vi "wrap.PullString.vi"(0 "class.GLue in":refnum<class "class.GLue.lvclass">, 11 "error in (no error)":errorcluster, 13 "Index":i32=-1) -> (4 "class.GLue out":refnum<class "class.GLue.lvclass">, 8 "String":string, 15 "error out":errorcluster)   [LabVIEW 2014, in "GLue.lvlib" / "class.GLue.lvclass"]
uses:
  class.GLue.lvclass
  class.GLue.lvclass/class.GLue.ctl
  Resources/GLue.dll
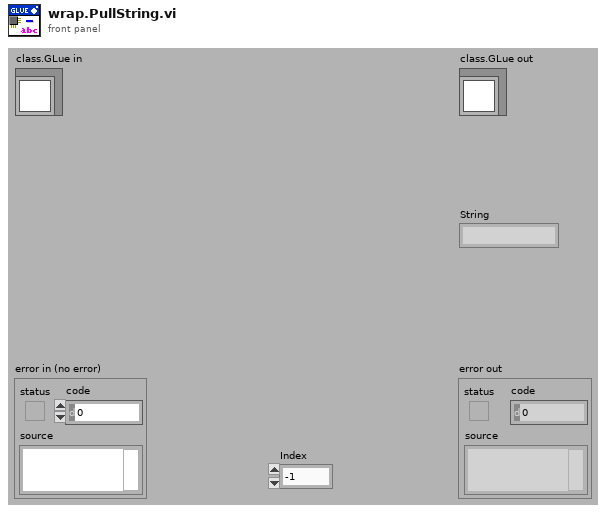
[diagram p1: front panel]
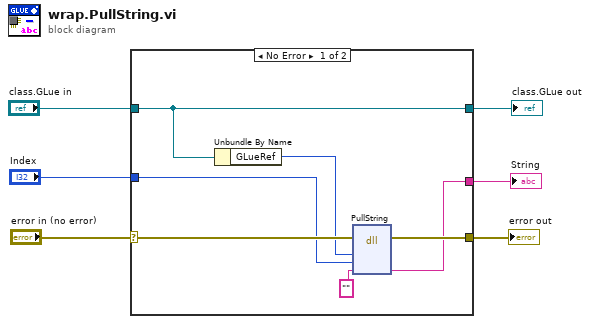
[diagram p0: block diagram]
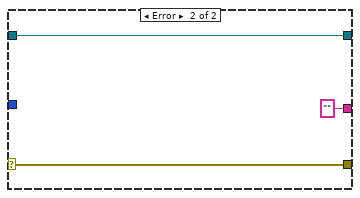
[diagram p2: hidden frame]
diagram:
  n1 = case shown="No Error" "error in (no error)" {
    selector: "error in (no error)" -> [w12 w16]
    tunnel: [w11 w16] -> w5
    tunnel: [w13 w15] -> w3
    tunnel: "class.GLue in" -> [w13 w15]
    tunnel: "Index" -> [w9 _]
    tunnel: [w8 "" ("String")] -> w1
    frame No Error {
      n2 = Unbundle By Name(w13) -> ("GLueRef"=w10:i64)
      n3 = dll-call lib="C:/Users/Antonie/Documents/work/glue/trunk/Resources/GLue.dll" fn="PullString"(error in=w12, "MLua"=w10, "Index"=w9, "String"="") -> (error out=w11:errorcluster, "String"=w8:string)  [unwired: 5 in, 1 out]
    }
    frame Error {
    }
  }
  "error out" <- w5
  "class.GLue out" <- w3
  "String" <- w1
